vi "Send MC Telemetry.vi"   [LabVIEW 2015]
uses:
  MC Telemetry.ctl
  MC Temp 1.ctl
  MC Temp 2.ctl
  MC Temp 3.ctl
  MC Current.ctl
  MC Voltage.ctl
  MC State.ctl
  Inverter States.ctl
  Inverter Run Modes.ctl
  VSM States.ctl
  MC Torque.ctl
  MC Position.ctl
  MC Faults.ctl
  MC Flux.ctl
  MC Internal Voltages.ctl
  MC Mod Index and Flux Weakening.ctl
  Global Data.vi
types:
  T1 = typedef "MC Telemetry.ctl" = cluster{"MC Temp 1":T2, "MC Temp 2":T3, "MC Temp 3":T4, "MC Current":T5, "MC Voltage":T6, "MC State":T7, "MC Torque":T11, "MC Position":T12, "MC Faults":T13, "MC Flux":T14, "MC Internal Voltages":T15, "Mod Index & Flux Weakening":T16}
  T2 = typedef "MC Temp 1.ctl" = cluster{"TMCModuleA":dbl, "TMCModuleB":dbl, "TMCModuleC":dbl, "TMCGateDriver":dbl}
  T3 = typedef "MC Temp 2.ctl" = cluster{"TMCControlBoard":dbl, "TMCRTD1":dbl, "TMCRTD2":dbl, "TMCRTD3":dbl}
  T4 = typedef "MC Temp 3.ctl" = cluster{"TMCRTD4":dbl, "TMCRTD5":dbl, "TMotor":dbl, "MTorqueShudder":dbl}
  T5 = typedef "MC Current.ctl" = cluster{"IMCPhaseA":dbl, "IMCPhaseB":dbl, "IMCPhaseC":dbl, "IMCBatteryCalc":dbl}
  T6 = typedef "MC Voltage.ctl" = cluster{"VMCPhaseAB":dbl, "VMCPhaseBC":dbl, "VMCOutput":dbl, "VMCBattery":dbl}
  T7 = typedef "MC State.ctl" = cluster{"eMCInverterState":T8, "eMCInverterRunMode":T9, "eMCInverterCommandMode":enum16{"CAN Mode", "VSM Mode"}, "bMCInverterEnable":bool, "bMCInverterEnableLockout":bool, "bMCDirectionForward":bool, "eMCVSMState":T10, "bMCRelay1":bool, "bMCRelay2":bool, "bMCRelay3":bool, "bMCRelay4":bool}
  T8 = typedef "Inverter States.ctl" = enum16{"Power On", "Stop", "Open Loop", "Closed Loop", "Wait", "Internal", "Idle Run", "Idle Stop", ""}
  T9 = typedef "Inverter Run Modes.ctl" = enum16{"Torque Mode", "Speed Mode"}
  T10 = typedef "VSM States.ctl" = enum16{"VSM Start", "Pre-Charge Init", "Pre-Charge Active", "Pre-Charge Complete", "VSM Wait", "VSM Ready", "Motor Running", "Blink Fault Code", "Shutdown in Process", "Recycle Power"}
  T11 = typedef "MC Torque.ctl" = cluster{"MMCRequested":dbl, "MMCFeedback":dbl, "tMCElapsed":u32}
  T12 = typedef "MC Position.ctl" = cluster{"aMotor":dbl, "nMotor":dbl, "fMCOutput":dbl, "aDeltaResolverFilt":dbl}
  T13 = typedef "MC Faults.ctl" = cluster{"MC Fault":cluster{"Over-Speed":bool, "Over-Current":bool, "Over-Voltage":bool, "Inverter Over-Temp":bool, "Direction Command":bool, "Inverter Response Time-Out":bool, "Desat Fault":bool, "Hardware Over-Current":bool, "Under-Voltage":bool, "CAN Command Message Lost":bool, "Motor Over-Temp":bool, "Module A Over-Temp":bool, "Module B Over-Temp":bool, "Module C Over-Temp":bool, "PCB Over-Temp":bool, "Gate Driver 1 Over-Temp":bool, "Gate Driver 2 Over-Temp":bool, "Gate Drive 3 Over-Temp":bool, "Current Sensor Fault":bool, "Resolver Not Connected":bool}, "MC Post":u32, "MC RUN":u32}
  T14 = typedef "MC Flux.ctl" = cluster{"IMCFluxCommand":dbl, "IMCFluxFeedback":dbl, "IMC_Id":dbl, "IMC_Iq":dbl}
  T15 = typedef "MC Internal Voltages.ctl" = cluster{"VMCRef1_5":dbl, "VMCRef2_5":dbl, "VMCRef5":dbl, "VMCRef12":dbl}
  T16 = typedef "MC Mod Index and Flux Weakening.ctl" = cluster{"NMCModulationIndex":dbl, "IMCFluxWeakeningOutput":dbl, "IMCIdCommand":dbl, "IMCIqCommand":dbl}
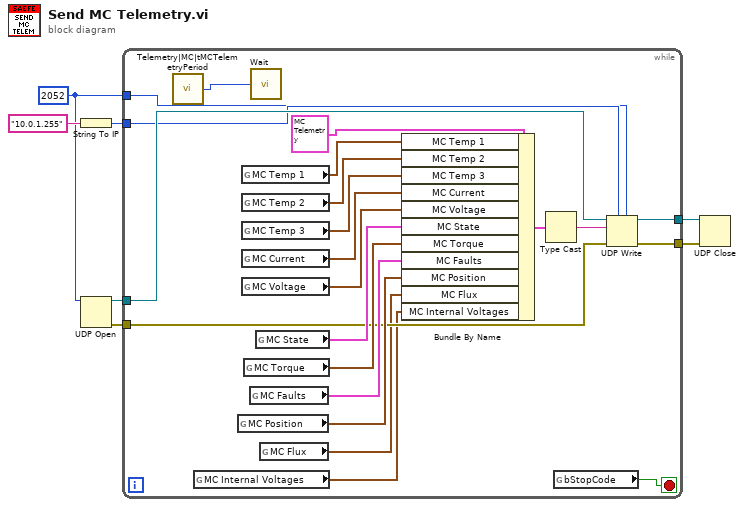
[diagram p0: block diagram]
diagram:
  w2 = u16 2052 ("port")
  n1 = String To IP(1:"10.0.1.255" ("name")) -> (0:w1:u32)
  n2 = UDP Open(11:w2) -> (port=w6:refnum<k16>, 0:w5:errorcluster)  [unwired: 4 in, 1 out]
  n3 = while {
    tunnel: w6 -> [w18]
    tunnel: w5 -> [w17]
    tunnel: [w14] -> w4
    tunnel: [w13] -> w3
    tunnel: w1 -> [w12]
    tunnel: w2 -> [w11]
    stop <- w29 stop-if-true
    n4 = call "Telemetry|MC|tMCTelemetryPeriod"() -> ("Value"=w8:u32)
    n5 = global read "Global Data.vi" "MC Internal Voltages"() -> (w9:T15)
    n6 = global read "Global Data.vi" "MC Position"() -> (w19:T12)
    n7 = global read "Global Data.vi" "MC Temp 1"() -> (w27:T2)
    n8 = global read "Global Data.vi" "MC Temp 2"() -> (w26:T3)
    n9 = global read "Global Data.vi" "MC Temp 3"() -> (w25:T4)
    n10 = global read "Global Data.vi" "MC Current"() -> (w24:T5)
    n11 = global read "Global Data.vi" "MC Voltage"() -> (w23:T6)
    n12 = global read "Global Data.vi" "MC Torque"() -> (w21:T11)
    n13 = global read "Global Data.vi" "MC Faults"() -> (w20:T13)
    n14 = call "Wait"("Count(mSec)"=w8) -> ()  [unwired: 1 out]
    n15 = global read "Global Data.vi" "MC State"() -> (w22:T7)
    n16 = global read "Global Data.vi" "MC Flux"() -> (w10:T14)
    n17 = Bundle By Name(cluster=T1 {"MC Temp 1"={"TMCModuleA"=0.0, "TMCModuleB"=0.0, "TMCModuleC"=0.0, "TMCGateDriver"=0.0}, "MC Temp 2"={"TMCControlBoard"=0.0, "TMCRTD1"=0.0, "TMCRTD2"=0.0, "TMCRTD3"=0.0}, "MC Temp 3"={"TMCRTD4"=0.0, "TMCRTD5"=0.0, "TMotor"=0.0, "MTorqueShudder"=0.0}, "MC Current"={"IMCPhaseA"=0.0, "IMCPhaseB"=0.0, "IMCPhaseC"=0.0, "IMCBatteryCalc"=0.0}, "MC Voltage"={"VMCPhaseAB"=0.0, "VMCPhaseBC"=0.0, "VMCOutput"=0.0, "VMCBattery"=0.0}, "MC State"={"eMCInverterState"=enum."Power On", "eMCInverterRunMode"=enum."Torque Mode", "eMCInverterCommandMode"=enum."CAN Mode", "bMCInverterEnable"=FALSE, "bMCInverterEnableLockout"=FALSE, "bMCDirectionForward"=FALSE, "eMCVSMState"=enum."VSM Start", "bMCRelay1"=FALSE, "bMCRelay2"=FALSE, "bMCRelay3"=FALSE, "bMCRelay4"=FALSE}, "MC Torque"={"MMCRequested"=0.0, "MMCFeedback"=0.0, "tMCElapsed"=0}, "MC Position"={"aMotor"=0.0, "nMotor"=0.0, "fMCOutput"=0.0, "aDeltaResolverFilt"=0.0}, "MC Faults"={"MC Fault"={"Over-Speed"=FALSE, "Over-Current"=FALSE, "Over-Voltage"=FALSE, "Inverter Over-Temp"=FALSE, "Direction Command"=FALSE, "Inverter Response Time-Out"=FALSE, "Desat Fault"=FALSE, "Hardware Over-Current"=FALSE, "Under-Voltage"=FALSE, "CAN Command Message Lost"=FALSE, "Motor Over-Temp"=FALSE, "Module A Over-Temp"=FALSE, "Module B Over-Temp"=FALSE, "Module C Over-Temp"=FALSE, "PCB Over-Temp"=FALSE, "Gate Driver 1 Over-Temp"=FALSE, "Gate Driver 2 Over-Temp"=FALSE, "Gate Drive 3 Over-Temp"=FALSE, "Current Sensor Fault"=FALSE, "Resolver Not Connected"=FALSE}, "MC Post"=0, "MC RUN"=0}, "MC Flux"={"IMCFluxCommand"=0.0, "IMCFluxFeedback"=0.0, "IMC_Id"=0.0, "IMC_Iq"=0.0}, "MC Internal Voltages"={"VMCRef1_5"=0.0, "VMCRef2_5"=0.0, "VMCRef5"=0.0, "VMCRef12"=0.0}, "Mod Index & Flux Weakening"={"NMCModulationIndex"=0.0, "IMCFluxWeakeningOutput"=0.0, "IMCIdCommand"=0.0, "IMCIqCommand"=0.0}} ("MC Telemetry"), "MC Temp 1"=w27, "MC Temp 2"=w26, "MC Temp 3"=w25, "MC Current"=w24, "MC Voltage"=w23, "MC State"=w22, "MC Torque"=w21, "MC Faults"=w20, "MC Position"=w19, "MC Flux"=w10, "MC Internal Voltages"=w9) -> (w16:T1)
    n18 = Type Cast(x=w16) -> (*(type *) &x=w15:string)  [unwired: 1 in]
    n19 = global read "Global Data.vi" "bStopCode"() -> (w29:bool)
    n20 = UDP Write(address=w12, port or service name=w11, connection ID=w18, data in=w15, 8:w17) -> (error out=w13:errorcluster, 3:w14:refnum<k16>)  [unwired: 1 in]
  }
  n21 = UDP Close(connection ID=w4, 8:w3) -> ()  [unwired: 2 out]
